vi "Set Bounds.vi"(8 "error in (no error)":errorcluster, 10 "Bounds":T1, 11 "IObject in":refnum<class "IObject.lvclass">) -> (0 "error out":errorcluster, 3 "IObject out":refnum<class "IObject.lvclass">)   [LabVIEW 2013, in "IObject.lvclass"]
uses:
  IObject.lvclass
  <vilib>/Utility/miscctls.llb/LVRectTypeDef.ctl
  IObject.lvclass/IObject.ctl
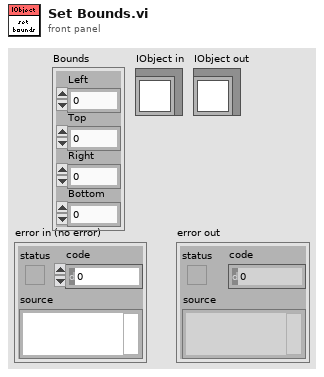
[diagram p1: front panel]
types:
  T1 = typedef "LVRectTypeDef.ctl" = cluster{"Left":i16, "Top":i16, "Right":i16, "Bottom":i16}
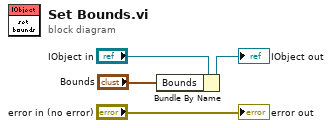
[diagram p0: block diagram]
diagram:
  n1 = Bundle By Name(cluster="IObject in", "Bounds"="Bounds") -> (→"IObject out":refnum<class "IObject.lvclass">)
  "error out" <- "error in (no error)"
